vi "Signal Simulator.vi"() -> ()   [LabVIEW 2017]
uses:
  <vilib>/Analysis/NI_AALBase.lvlib
panel:
  in  "Sampling Rate":dbl=1.0 format="%#_p"
  out "FFT Gain":dbl
  out "Noise (W|50ohms)":dbl
  out "k":dbl
  out "Noise vrms":dbl
  in  "Desired SNR (dB)":dbl=80.0 format="%#_p"
  in  "Oscillator Magnitude":dbl=1.0 format="%#_13g"
  in  "Oscillator Frequency":dbl=0.001 format="%#_p"
  in  "Signal Offset":cdb format="%#_13g"
  in  "Singal Amplitude":dbl=1.0 format="%#_13g"
  in  "Signal Frequency":dbl=0.001 format="%#_p"
  in  "Number Samples":i32=8192
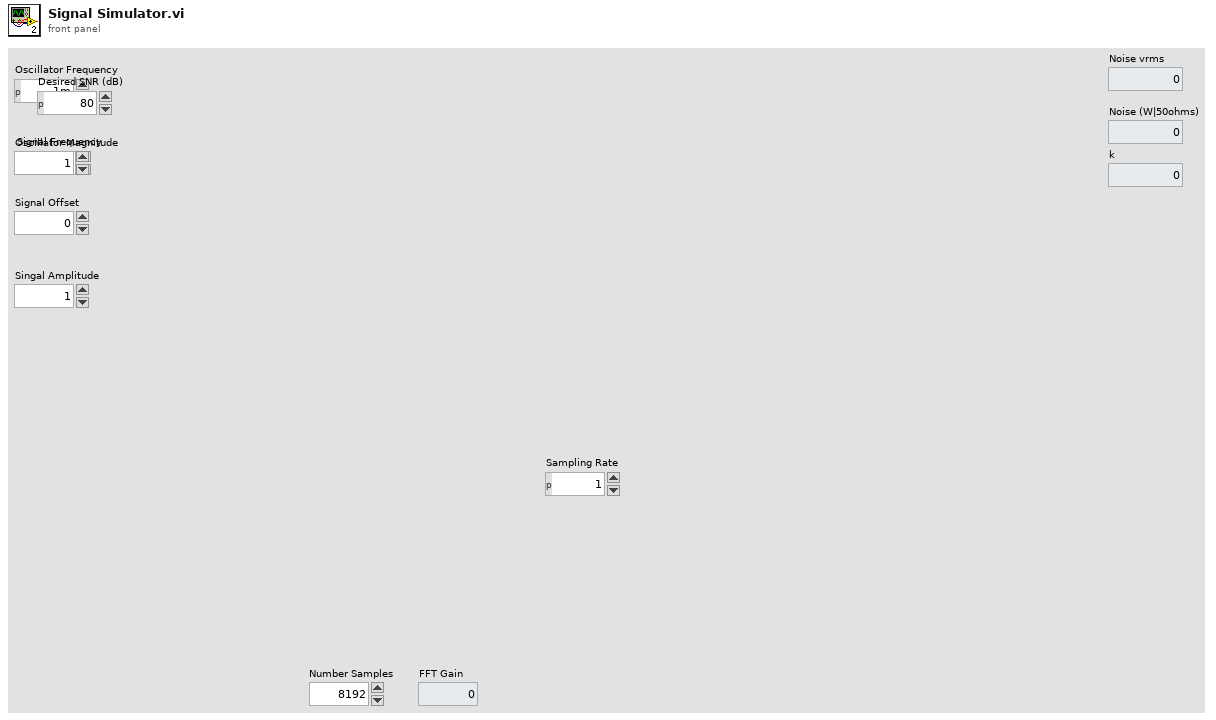
[diagram p1: front panel]
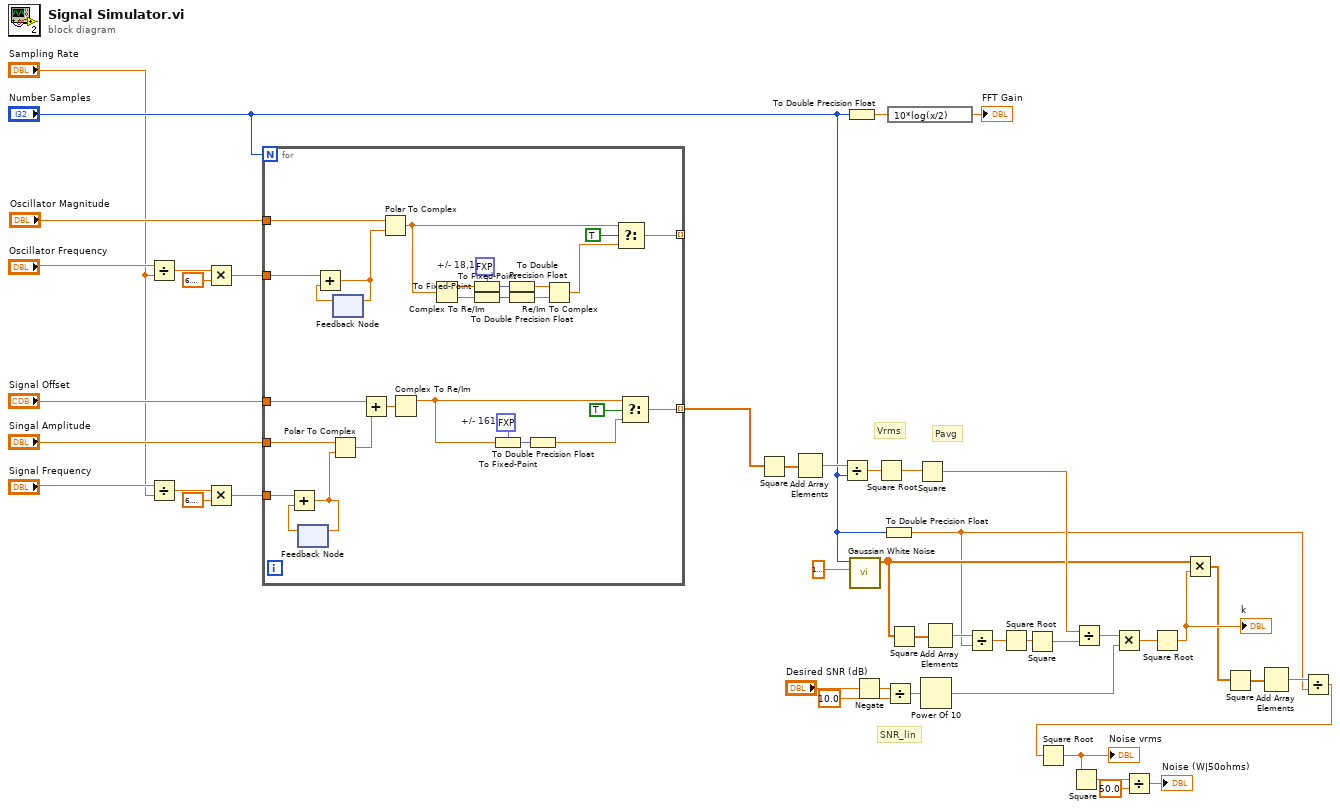
[diagram p0: block diagram]
diagram:
  # "SNR_lin"
  # "Pavg"
  # "Vrms"
  n1 = Divide(x="Oscillator Frequency", y="Sampling Rate") -> (x/y=w39:dbl)
  n2 = Divide(x="Signal Frequency", y="Sampling Rate") -> (x/y=w43:dbl)
  n3 = Multiply(x=w39, y=6.283185307179586) -> (x*y=w36:dbl)
  n4 = Multiply(x=w43, y=6.283185307179586) -> (x*y=w42:dbl)
  n5 = for {
    N: "Number Samples" -> [_]
    tunnel: w42 -> [w69]
    tunnel: "Singal Amplitude" -> [w72]
    tunnel: "Signal Offset" -> [w71]
    tunnel: [w55] -> _ mode=indexing
    tunnel: [w49] -> w2 mode=indexing
    tunnel: w36 -> [w60]
    tunnel: "Oscillator Magnitude" -> [w58]
    w50 = fxp<+/-,16,1> 0.0  # +/- 161
    w65 = fxp<+/-,18,1> 0.0  # +/- 18,1
    n6 = feedback #1() -> (w73:dbl)  [unwired: 1 in]
    n7 = Add(x=w69, y=w73) -> (x+y=w68:dbl)
    n8 = feedback-in #1(w68) -> ()
    n9 = Polar To Complex(1:w68, 2:w72) -> (0:w70:cdb)
    n10 = feedback #2() -> (w59:dbl)  [unwired: 1 in]
    n11 = Add(x=w60, y=w59) -> (x+y=w57:dbl)
    n12 = feedback-in #2(w57) -> ()
    n13 = Add(x=w71, y=w70) -> (x+y=w47:cdb)
    n14 = Polar To Complex(1:w57, 2:w58) -> (0:w56:cdb)
    n15 = Complex To Re/Im(x + iy=w47) -> (x=w46:dbl)  [unwired: 1 out]
    n16 = Complex To Re/Im(x + iy=w56) -> (x=w67:dbl, y=w66:dbl)
    n17 = To Fixed-Point(fixed-point type=w65, number=w67) -> (fixed-point=w64:fxp<+/-,18,1>)
    n18 = To Fixed-Point(fixed-point type=w65, number=w66) -> (fixed-point=w63:fxp<+/-,18,1>)
    n19 = To Fixed-Point(fixed-point type=w50, number=w46) -> (fixed-point=w51:fxp<+/-,16,1>)
    n20 = To Double Precision Float(number=w64) -> (double precision float=w62:dbl)
    n21 = To Double Precision Float(number=w63) -> (double precision float=w61:dbl)
    n22 = To Double Precision Float(number=w51) -> (double precision float=w48:dbl)
    n23 = Re/Im To Complex(1:w61, 2:w62) -> (0:w54:cdb)
    n24 = Select(t=w56, s=TRUE, f=w54) -> (s? t:f=w55:cdb)
    n25 = Select(t=w46, s=TRUE, f=w48) -> (s? t:f=w49:dbl)
  }
  n26 = Square(x=w2) -> (x^2=w34:dbl[])
  n27 = Add Array Elements(numeric array=w34) -> (sum=w33:dbl)
  n28 = Divide(x=w33, y="Number Samples") -> (x/y=w32:dbl)
  n29 = To Double Precision Float(number="Number Samples") -> (double precision float=w5:dbl)
  n30 = call <vilib>:"Gaussian White Noise.vi"("standard deviation"=1.0000000000000002, "samples"="Number Samples") -> ("Gaussian noise pattern"=w16:dbl[])  [unwired: 8 in, 1 out]
  n31 = Negate(x="Desired SNR (dB)") -> (-x=w19:dbl)
  n32 = Square Root(x=w32) -> (sqrt(x)=w31:dbl)
  n33 = To Double Precision Float(number="Number Samples") -> (double precision float=w3:dbl)
  n34 = Divide(x=w19, y=10.0) -> (x/y=w27:dbl)
  n35 = expression code="10*log(x/2)"(w5) -> (→"FFT Gain":dbl)
  n36 = Square(x=w16) -> (x^2=w23:dbl[])
  n37 = Square(x=w31) -> (x^2=w22:dbl)
  n38 = Power Of 10(x=w27) -> (10^x=w18:dbl)
  n39 = Add Array Elements(numeric array=w23) -> (sum=w24:dbl)
  n40 = Divide(x=w24, y=w3) -> (x/y=w25:dbl)
  n41 = Square Root(x=w25) -> (sqrt(x)=w26:dbl)
  n42 = Square(x=w26) -> (x^2=w21:dbl)
  n43 = Divide(x=w22, y=w21) -> (x/y=w20:dbl)
  n44 = Multiply(x=w20, y=w18) -> (x*y=w17:dbl)
  n45 = Square Root(x=w17) -> (sqrt(x)=w15:dbl)
  "k" <- w15
  n46 = Multiply(x=w16, y=w15) -> (x*y=w7:dbl[])
  n47 = Square(x=w7) -> (x^2=w14:dbl[])
  n48 = Add Array Elements(numeric array=w14) -> (sum=w13:dbl)
  n49 = Divide(x=w13, y=w3) -> (x/y=w12:dbl)
  n50 = Square Root(x=w12) -> (sqrt(x)=w11:dbl)
  "Noise vrms" <- w11
  n51 = Square(x=w11) -> (x^2=w10:dbl)
  n52 = Divide(x=w10, y=50.0) -> (x/y=→"Noise (W|50ohms)":dbl)
